vi "Namen fuer LIN MG File erzeugen.vi"(11 "String Eingabe":T1) -> (2 "EPA TXT Datei Name":string, 3 "LIN TXT Datei Name":string)   [LabVIEW 2020, in "Linearisierung v2.lvlib"]
uses:
  Linearisierung v2.lvlib
  Visualisierungs Elemente/String - Eingabefeld.ctl
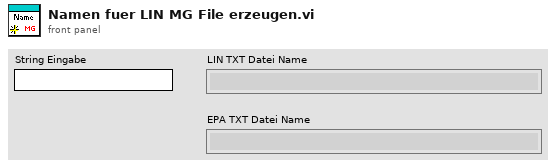
[diagram p1: front panel]
types:
  T1 = typedef "String - Eingabefeld.ctl" = string
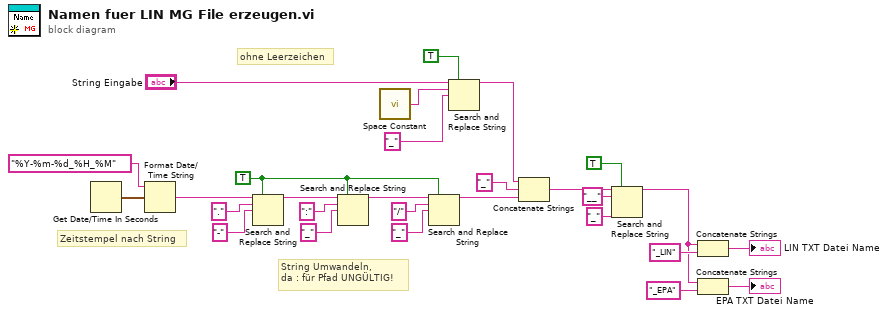
[diagram p0: block diagram]
diagram:
  w17 = TRUE ("Alle ersetzen? (F)")
  # "ohne Leerzeichen"
  # "String Umwandeln, \nda : für Pfad UNGÜLTIG!"
  # "Zeitstempel nach String"
  n1 = Get Date/Time In Seconds() -> (seconds since 1Jan1904=w28:timestamp)
  n2 = Format Date/Time String(time format string (%c)="%Y-%m-%d_%H_%M" ("Zeitformatierungs-String (%c)"), seconds (now)=w28) -> (date/time string=w27:string)  [unwired: 1 in]
  n3 = Search and Replace String(replace all?=w17, input string=w27, search string="." ("Such-String"), replace string="-" ("String ersetzen(\"\")")) -> (result string=w24:string)  [unwired: 4 in, 3 out]
  n4 = Search and Replace String(replace all?=w17, input string=w24, search string=":" ("Such-String"), replace string="_" ("String ersetzen(\"\")")) -> (result string=w18:string)  [unwired: 4 in, 3 out]
  n5 = call <vilib>:"Space Constant.vi"() -> ("String"=w10:string)
  n6 = Search and Replace String(replace all?=w17, input string=w18, search string="/" ("Such-String"), replace string="_" ("String ersetzen(\"\")")) -> (result string=w16:string)  [unwired: 4 in, 3 out]
  n7 = Search and Replace String(replace all?=TRUE ("Alle ersetzen? (F)"), input string="String Eingabe", search string=w10, replace string="_") -> (result string=w11:string)  [unwired: 4 in, 3 out]
  n8 = Concatenate Strings(w11, "_", w16) -> (w3:string)
  n9 = Search and Replace String(replace all?=TRUE ("Alle ersetzen? (F)"), input string=w3, search string="__" ("Such-String"), replace string="_" ("Ersetzungs-String (\"\")")) -> (result string=w2:string)  [unwired: 4 in, 3 out]
  n10 = Concatenate Strings(w2, "_LIN" ("String")) -> (→"LIN TXT Datei Name":string)
  n11 = Concatenate Strings(w2, "_EPA" ("String")) -> (→"EPA TXT Datei Name":string)
